vi "Core.vi"(0 "VI Reference In":refnum<vi>, 1 "Label":string, 2 "delimiter (>>)":string=">>", 3 "Assert Only? (F)":bool, 5 "Control Path":string, 7 "Disabled":T1(ring), 11 "Error In":errorcluster, 12 "Assert Interval(10 ms)":u32=10, 13 "Timeout(5 sec)":dbl=5.0) -> (4 "VI Reference Out":refnum<vi>, 6 "Test Control State":T1(ring), 15 "Error Out":errorcluster)   [LabVIEW 2016, in "Drona.lvlib" / "AssertControlDisable.lvlib"]
doc: "Asserts the state of controls.\n\nThe input control name is given as a string , incase of path, use delimiters inbetween the path."
uses:
  AssertControlDisable.lvlib
  Get/GetControlRef/GetControlRefByPath.vi
  <vilib>/addons/_JKI Toolkits/Caraya/classes/Assert/Assert Equal Value_Variant.vi
  <vilib>/addons/_JKI Toolkits/Caraya/classes/Assert/Assert.lvclass
  Get/GetControlRef/GetControlRef.lvlib
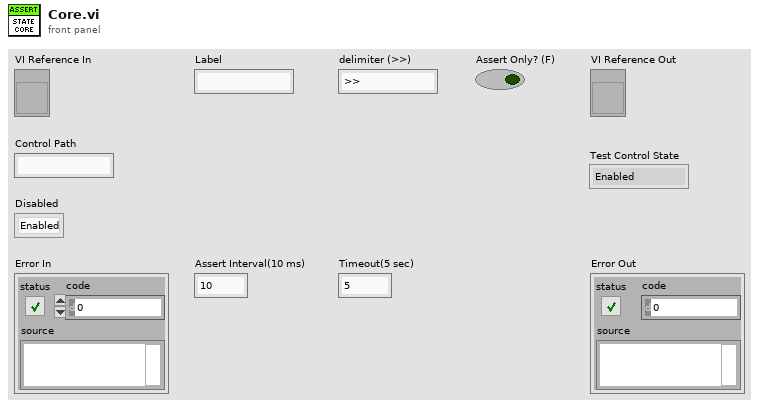
[diagram p1: front panel]
types:
  T1 = enum8{"Enabled", "Disabled", "Disabled and Grayed Out"}
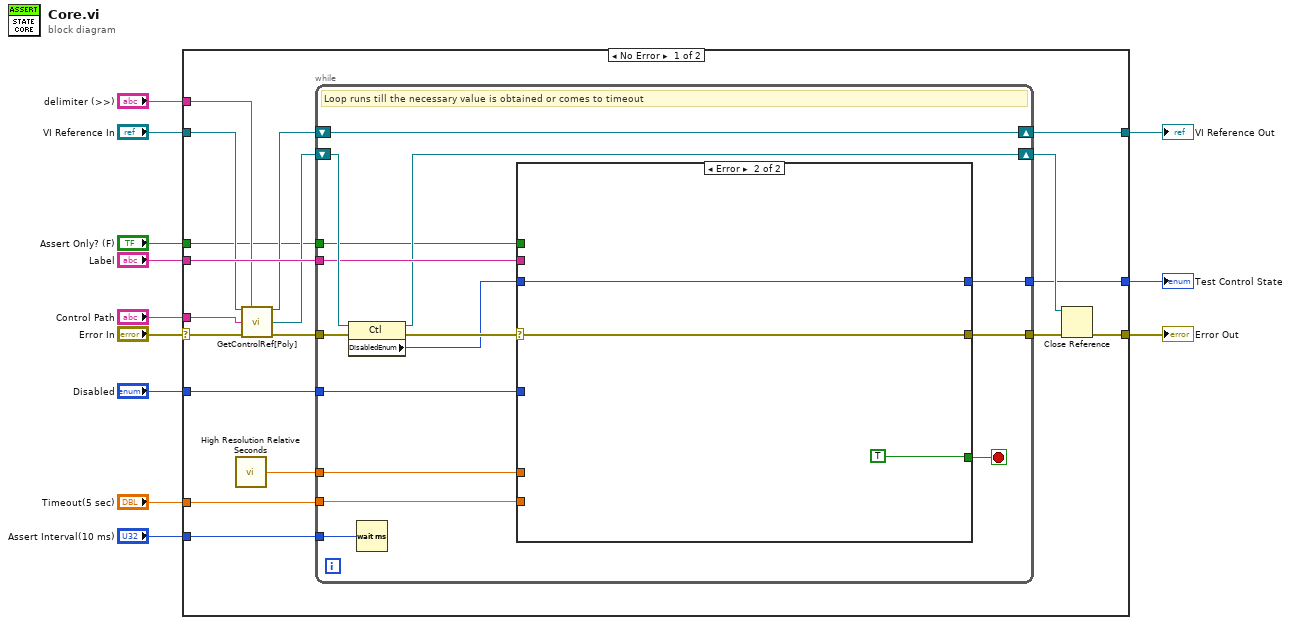
[diagram p0: block diagram]
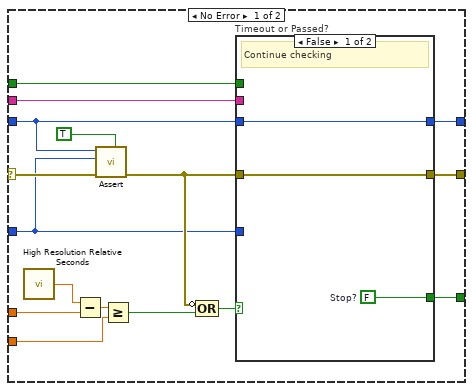
[diagram p2: hidden frame]
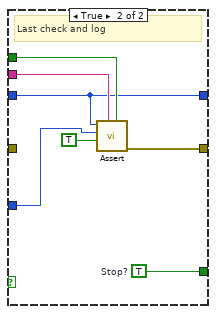
[diagram p3: hidden frame]
diagram:
  n1 = case shown="No Error" "Error In" {
    selector: "Error In" -> [w25 w76]
    tunnel: "Timeout(5 sec)" -> [w30 _]
    tunnel: [w29 w75] -> w11
    tunnel: [w18 w76] -> w10
    tunnel: "Assert Interval(10 ms)" -> [w27 _]
    tunnel: "Label" -> [w26 _]
    tunnel: "VI Reference In" -> [w24 w75]
    tunnel: "Control Path" -> [w23 _]
    tunnel: "delimiter (>>)" -> [w16 _]
    tunnel: "Assert Only? (F)" -> [w15 _]
    tunnel: "Disabled" -> [w14 _]
    tunnel: [w13 _] -> w1
    frame No Error {
      n2 = call <vilib>:"High Resolution Relative Seconds.vi"() -> ("relative seconds"=w22:dbl)
      n3 = call-poly "GetControlRef[Poly].vi"("VI Reference In"=w24, "delimiter (>>)"=w16, "Control Path"=w23, "error In"=w25) -> ("VI Reference Out"=w20:refnum<vi>, "Ctl Refnum"=w19:refnum<vi>, "error out"=w21:errorcluster)  [unwired: 9 in]
      n4 = while {
        tunnel: w30 -> [w44]
        tunnel: w22 -> [w45]
        tunnel: w21 -> [w39]
        tunnel: [w42] -> w28
        tunnel: w27 -> [w40]
        tunnel: w26 -> [w36]
        shift-right: [w37] -> w29
        shift-left: w20 -> [w37]
        shift-right: [w35] -> w17
        shift-left: w19 -> [w38]
        tunnel: w15 -> [w34]
        tunnel: w14 -> [w32]
        tunnel: [w31] -> w13
        stop <- w43 stop-if-true
        # "Loop runs till the necessary value is obtained or comes to timeout"
        n5 = property class="Ctl"(reference=w38, error in=w39) -> (reference out=w35:refnum<vi>, error out=w41:errorcluster, "DisabledEnum"=w33:T1)
        n6 = Wait (ms)(milliseconds to wait=w40) -> ()  [unwired: 1 out]
        n7 = case shown="Error" w41 {
          selector: w41 -> [w57 w74]
          tunnel: w45 -> [w61 _]
          tunnel: w44 -> [w58 _]
          tunnel: [w50 TRUE] -> w43
          tunnel: [w51 w74] -> w42
          tunnel: w33 -> [w49 w72]
          tunnel: w36 -> [w56 _]
          tunnel: w34 -> [w48 _]
          tunnel: w32 -> [w47 _]
          tunnel: [w46 w72] -> w31
          frame No Error {
            n8 = call <vilib>:"High Resolution Relative Seconds.vi"() -> ("relative seconds"=w60:dbl)
            n9 = Subtract(x=w60, y=w61) -> (x-y=w59:dbl)
            n10 = call-poly <vilib>:"Assert.vi"("Assert Only? (F)"=TRUE, "error in (no error)"=w57, "Y"=w47, "X"=w49) -> ("error out"=w54:errorcluster)  [unwired: 7 in]
            n11 = Greater Or Equal?(x=w59, y=w58) -> (x >= y?=w55:bool)
            n12 = Compound Arithmetic op=OR(invert w54, w55) -> (w53:bool)
            n13 = case "Timeout or Passed?" shown="False" w53 {
              tunnel: w54 -> [w64 _]
              tunnel: w49 -> [w62 w65]
              tunnel: w56 -> [_ w71]
              tunnel: [w64 w70] -> w51
              tunnel: [w63 w69] -> w50
              tunnel: w48 -> [_ w67]
              tunnel: w47 -> [_ w66]
              tunnel: [w62 w65] -> w46
              frame False {
                w63 = FALSE  # Stop?
                # "Continue checking"
              }
              frame True {
                w69 = TRUE  # Stop?
                # "Last check and log"
                n14 = call-poly <vilib>:"Assert.vi"("Assert Only? (F)"=w67, "Label"=w71, "Register with caller test (F)"=TRUE, "Y"=w66, "X"=w65) -> ("error out"=w70:errorcluster)  [unwired: 6 in]
              }
            }
          }
          frame Error {
          }
        }
      }
      n15 = Close Reference(reference=w17, error in (no error)=w28) -> (error out=w18:errorcluster)
    }
    frame Error {
    }
  }
  "Error Out" <- w10
  "VI Reference Out" <- w11
  "Test Control State" <- w1
